vi "weight_experimental1.vi"(10 "N_points":i32=4200, 11 "PV weight":dbl caption="g" format="%#.0f") -> (1 "Q3":dbl caption="mg/s" format="%#.0f", 2 "Q 1":dbl caption="mg/s" format="%#.0f", 3 "Weight 1":dbl caption="g" format="%#.0f", 5 "This VI":refnum<vi>)   [LabVIEW 2019]
uses:
  <vilib>/Analysis/baseanly.llb/Mean (DBL).vi
  <vilib>/Analysis/NI_AALBase.lvlib
panel:
  in  "Tab Control":T1(tab)
  out "dM 3":dbl caption="g" format="%#.0f"
  out "dM 1":dbl caption="g" format="%#.0f"
  out "variance":dbl format="%0.2f"
  out "standard deviation":dbl format="%0.2f"
  in  "Tare":dbl caption="g" format="%#.0f"
  in  "<0>":bool
  in  "<вес>":bool
  in  "k":dbl=1.0 caption="g" format="%#.3f"
  in  "Вес":dbl caption="g" format="%#.0f"
  # "Усреднение за 1 мин"
  # "(расход)"
  # "Усреднение за 3 мин"
  # "(расход)"
  # "Вес тары\n(полностью очистить бункер от продукта\nи запомнить PV weight или ввести вручную)."
  # "Вес тары\n(ввести фактический вес без учета тары\nили ввести k вручную)"
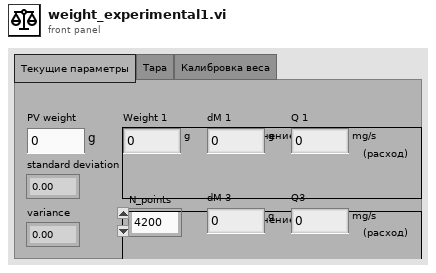
[diagram p1: front panel]
types:
  T1 = enum32{"Текущие параметры", "Тара", "Калибровка веса"}
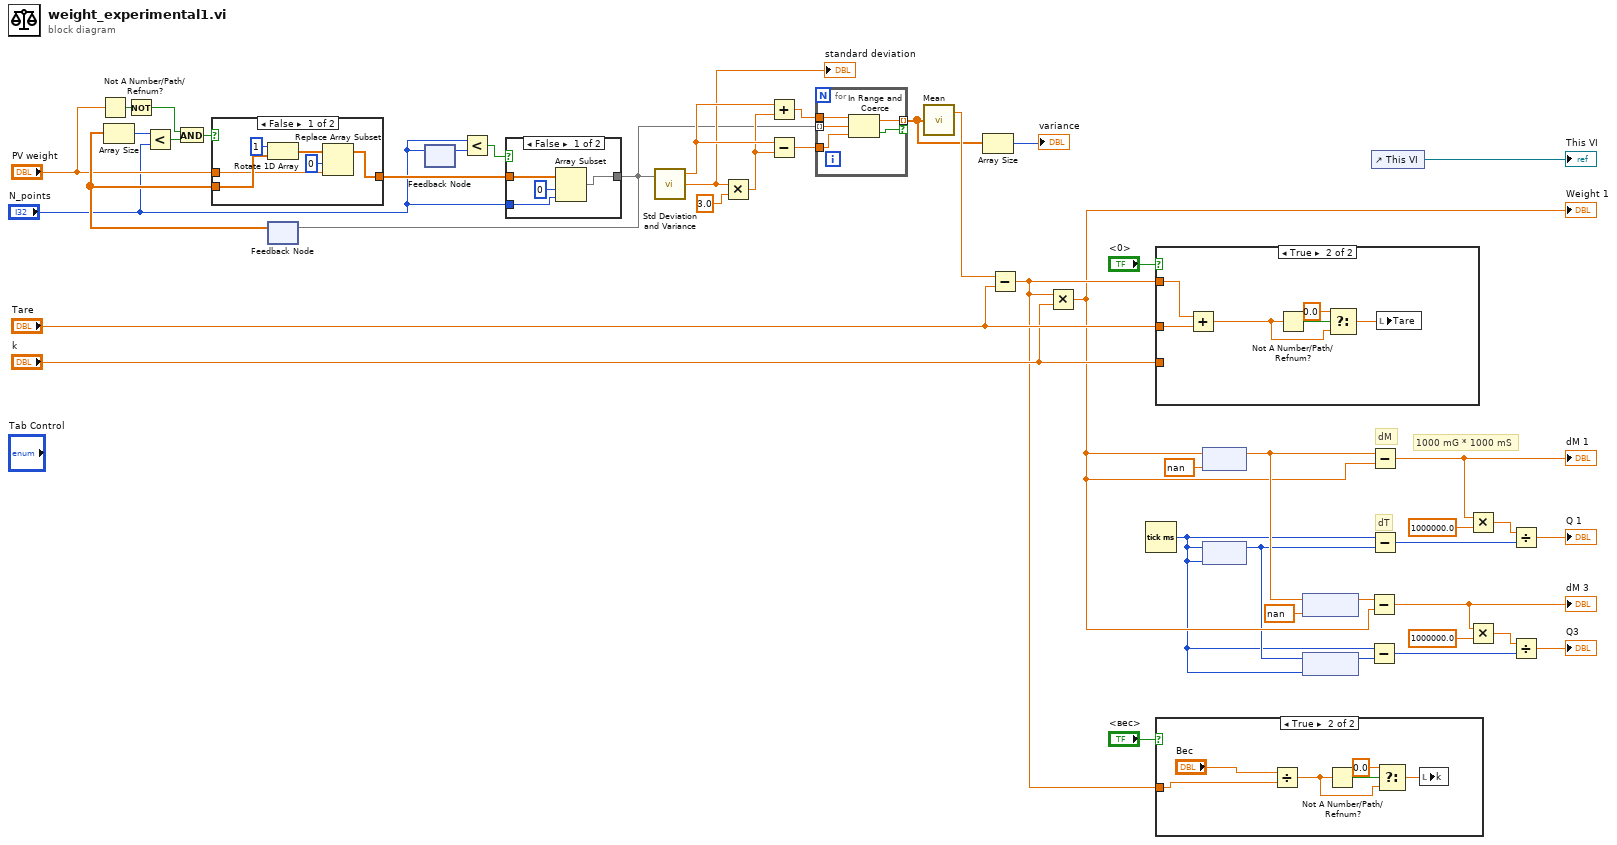
[diagram p0: block diagram]
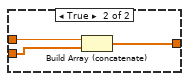
[diagram p3: hidden frame]
diagram:
  # "1000 mG * 1000 mS"
  # "dM"
  # "dT"
  n1 = Not A Number/Path/Refnum?(number/path/refnum="PV weight") -> (NaN/Path/Refnum?=w8:bool)
  n2 = Not(x=w8) -> (.not. x?=w6:bool)
  n3 = feedback #1() -> (w11:dbl[])  [unwired: 1 in]
  n4 = Array Size(array=w11) -> (size(s)=w12:i32)
  n5 = Less?(x=w12, y="N_points") -> (x < y?=w10:bool)
  n6 = And(x=w6, y=w10) -> (x .and. y?=w9:bool)
  n7 = case shown="False" w9 {
    tunnel: [w46 w53] -> w5
    tunnel: "PV weight" -> [w47 w54]
    tunnel: w11 -> [w48 w52]
    frame False {
      n8 = Rotate 1D Array(1:w48, 2:1 ("n")) -> (0:w50:dbl[])
      n9 = Replace Array Subset(array=w50, new element=w47, index=0) -> (w46:dbl[])
    }
    frame True {
      n10 = Build Array (concatenate)(w54, w52) -> (w53:dbl[])
    }
  }
  n11 = feedback #2() -> (w3:i32)  [unwired: 1 in]
  n12 = feedback-in #2("N_points") -> ()
  n13 = Less?(x="N_points", y=w3) -> (x < y?=w2:bool)
  n14 = case shown="False" w2 {
    tunnel: [w57 w59] -> w1
    tunnel: w5 -> [w58 w59]
    tunnel: "N_points" -> [w55 _]
    frame False {
      n15 = Array Subset(array=w58, index=0, length=w55) -> (w57:dbl[])
    }
    frame True {
    }
  }
  n16 = feedback-in #1(w1) -> ()
  n17 = call <vilib>:"Std Deviation and Variance.vi"("X"=w1) -> ("mean"=w21:dbl, "standard deviation"=w15:dbl)  [unwired: 1 in, 1 out]
  "standard deviation" <- w15
  n18 = Multiply(x=w15, y=3.0) -> (x*y=w13:dbl)
  n19 = Add(x=w21, y=w13) -> (x+y=w20:dbl)
  n20 = Subtract(x=w21, y=w13) -> (x-y=w19:dbl)
  n21 = for {
    tunnel: w1 -> [w62] mode=indexing
    tunnel: w20 -> [w64]
    tunnel: w19 -> [w63]
    tunnel: [w61] -> w16 mode=indexing if=w60
    n22 = In Range and Coerce(upper limit=w64, x=w62, lower limit=w63) -> (coerced(x)=w61:dbl, In Range?=w60:bool)
  }
  n23 = call-poly <vilib>:"Mean.vi"("X"=w16) -> ("mean"=w18:dbl)  [unwired: 1 out]
  n24 = Array Size(array=w16) -> (size(s)=→"variance":i32)
  n25 = Subtract(x=w18, y="Tare") -> (x-y=w32:dbl)
  n26 = Multiply(x=w32, y="k") -> (x*y=w30:dbl)
  "Weight 1" <- w30
  n27 = Tick Count (ms)() -> (millisecond timer value=w27:u32)
  n28 = case shown="True" "<0>" {
    tunnel: "Tare" -> [_ w67]
    tunnel: w32 -> [_ w66]
    tunnel: "k" -> [_ _]
    frame False {
    }
    frame True {
      n29 = Add(x=w66, y=w67) -> (x+y=w65:dbl)
      n30 = Not A Number/Path/Refnum?(number/path/refnum=w65) -> (NaN/Path/Refnum?=w70:bool)
      n31 = Select(t=0.0 ("y"), s=w70, f=w65) -> (s? t:f=w68:dbl)
      n32 = local write "Tare"(w68) -> ()
    }
  }
  n33 = case shown="True" "<вес>" {
    tunnel: w32 -> [_ w71]
    frame False {
    }
    frame True {
      n34 = Divide(x="Вес", y=w71) -> (x/y=w74:dbl)
      n35 = Not A Number/Path/Refnum?(number/path/refnum=w74) -> (NaN/Path/Refnum?=w76:bool)
      n36 = Select(t=0.0 ("y"), s=w76, f=w74) -> (s? t:f=w73:dbl)
      n37 = local write "k"(w73) -> ()
    }
  }
  n38 = feedback #3(nan) -> (w41:dbl)
  n39 = feedback-in #3(w30) -> ()
  n40 = feedback #4(w27) -> (w29:u32)
  n41 = feedback-in #4(w27) -> ()
  n42 = feedback #5(nan) -> (w42:dbl)
  n43 = feedback-in #5(w41) -> ()
  n44 = feedback #6(w27) -> (w28:u32)
  n45 = feedback-in #6(w29) -> ()
  n46 = Subtract(x=w42, y=w30) -> (x-y=w23:dbl)
  "dM 3" <- w23
  n47 = Subtract(x=w27, y=w28) -> (x-y=w24:u32)
  n48 = Subtract(x=w41, y=w30) -> (x-y=w36:dbl)
  "dM 1" <- w36
  n49 = Subtract(x=w27, y=w29) -> (x-y=w34:u32)
  n50 = control-ref of="This VI"() -> (→"This VI":refnum<vi>)
  n51 = Multiply(x=w36, y=1000000.0) -> (x*y=w35:dbl)
  n52 = Multiply(x=w23, y=1000000.0) -> (x*y=w26:dbl)
  n53 = Divide(x=w35, y=w34) -> (x/y=→"Q 1":dbl)
  n54 = Divide(x=w26, y=w24) -> (x/y=→"Q3":dbl)
